vi "linspace (dbl).vi"(6 "interval type":T1(ring), 9 "n":i32=100, 10 "b":i16, 11 "a":i16) -> (3 "array":i16[](array[numeric]))   [LabVIEW 2010, in "common.lvlib"]
uses:
  common.lvlib
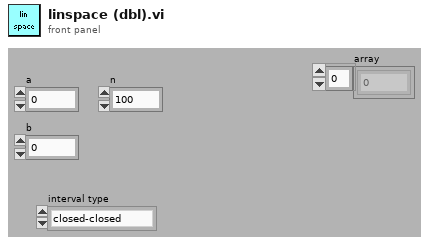
[diagram p1: front panel]
types:
  T1 = enum16{"closed-closed", "open-closed", "closed-open", "open-open"}
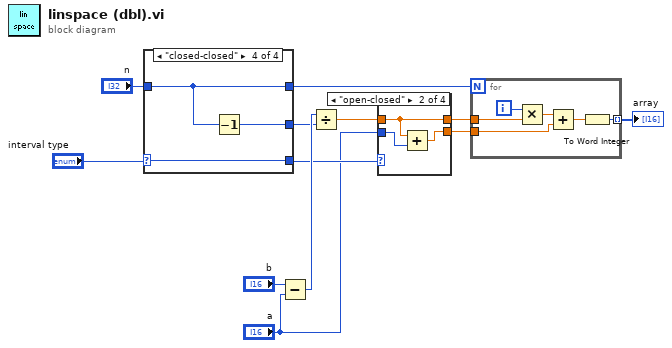
[diagram p0: block diagram]
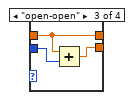
[diagram p3: hidden frame]
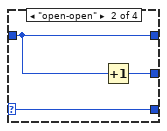
[diagram p6: hidden frame]
diagram:
  n1 = case shown="\"closed-closed\"" "interval type" {
    selector: "interval type" -> [w13 w15 w18 w20]
    tunnel: "n" -> [w14 w17 w19 w22]
    tunnel: [w14 w16 w19 w21] -> w8
    tunnel: [w14 w17 w19 w22] -> w7
    tunnel: [w13 w15 w18 w20] -> w5
    frame "open-closed" {
    }
    frame "open-open" {
      n2 = Increment(x=w17) -> (x+1=w16:i32)
    }
    frame "closed-open" {
    }
    frame "closed-closed" {
      n3 = Decrement(x=w22) -> (x-1=w21:i32)
    }
  }
  n4 = Subtract(x="b", y="a") -> (x-y=w11:i16)
  n5 = Divide(x=w11, y=w8) -> (x/y=w4:dbl)
  n6 = case shown="\"open-closed\"" w5 {
    tunnel: w4 -> [w23 w25 w28 w32]
    tunnel: "a" -> [w24 w27 w30 w31]
    tunnel: [w24 w26 w29 w31] -> w2
    tunnel: [w23 w25 w28 w32] -> w1
    frame "closed-closed", Default {
    }
    frame "open-closed" {
      n7 = Add(x=w25, y=w27) -> (x+y=w26:dbl)
    }
    frame "open-open" {
      n8 = Add(x=w28, y=w30) -> (x+y=w29:dbl)
    }
    frame "closed-open" {
    }
  }
  n9 = for {
    N: w7 -> [_]
    tunnel: w1 -> [w38]
    tunnel: w2 -> [w35]
    tunnel: [w33] -> w6 mode=indexing
    i -> [w37]
    n10 = Multiply(x=w37, y=w38) -> (x*y=w36:dbl)
    n11 = Add(x=w36, y=w35) -> (x+y=w34:dbl)
    n12 = To Word Integer(number=w34) -> (16bit integer=w33:i16)
  }
  "array" <- w6
